vi "_convertDataPluginInfoToItems.vi"(8 "error in (no error)":errorcluster, 11 "DataPlugin information":T1[](array[typedef])) -> (0 "error out":errorcluster, 3 "Items":string[][](array[string]))   [LabVIEW 2020]
uses:
  <vilib>/Platform/storage/utility/DataPluginSynchronization/_DataPluginInfo.ctl
  <vilib>/Platform/storage/utility/DataPluginSynchronization/_localizeDataPluginMessageEnum.ctl
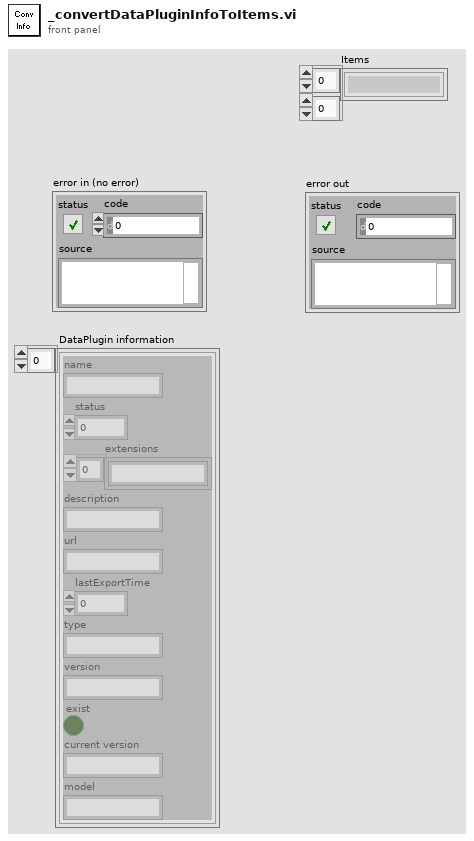
[diagram p1: front panel]
types:
  T1 = typedef "_DataPluginInfo.ctl" = cluster{"name":string, "status":u32, "extensions":string[], "description":string, "url":string, "lastExportTime":i64, "type":string, "version":string, "exist":bool, "current version":string, "model":string}
  T2 = typedef "_localizeDataPluginMessageEnum.ctl" = enum16{"Installed", "Not Installed", "Updates Available", "Latest version:", "Double click the \"Description\" cell.", "Install/Update DataPlugins", "Offline: ", "Please ensure that your network connection is working.", "No DataPlugins can be updated.", "Loading DataPlugins from ni.com/dataplugins", "Acquiring and installing ", "Install", "Update", "Succeed", "Failed", " Installation successful.", "Include *. to search for a file extension", "Current version:", " Installation failed.", "Installing update", "Update successful.", "Update failed.", "Updated", "Failed to update DataPlugins."}
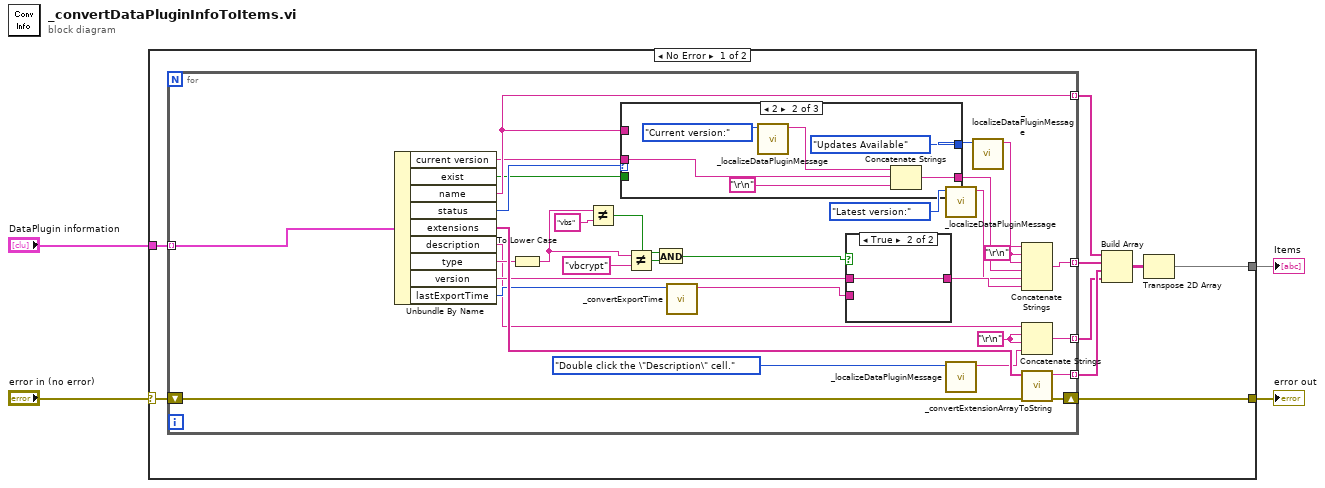
[diagram p0: block diagram]
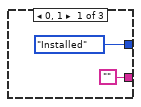
[diagram p3: hidden frame]
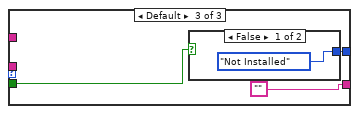
[diagram p4: hidden frame]
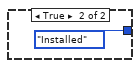
[diagram p5: hidden frame]
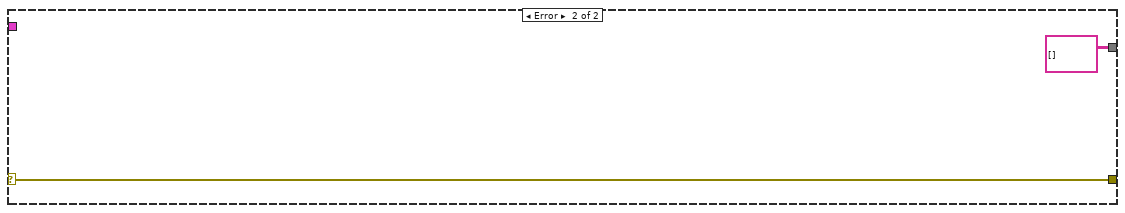
[diagram p6: hidden frame]
diagram:
  n1 = case shown="No Error" "error in (no error)" {
    selector: "error in (no error)" -> [w7 w62]
    tunnel: "DataPlugin information" -> [w5 _]
    tunnel: [w8 string[][] []] -> w4
    tunnel: [w6 w62] -> w2
    frame No Error {
      n2 = for {
        tunnel: w5 -> [w45] mode=indexing
        tunnel: [w18] -> w13 mode=indexing
        tunnel: [w28] -> w12 mode=indexing
        tunnel: [w43] -> w11 mode=indexing
        shift-right: [w41] -> w6
        shift-left: w7 -> [w42]
        tunnel: [w25] -> w10 mode=indexing
        w27 = "\r\n" ("string")
        w30 = "\r\n" ("string")
        n3 = Unbundle By Name(w45) -> ("current version"=w15:string, "exist"=w16:bool, "name"=w18:string, "status"=w40:u32, "extensions"=w44:string[], "description"=w26:string, "type"=w33:string, "version"=w32:string, "lastExportTime"=w39:i64)
        n4 = To Lower Case(string=w33) -> (all lower case string=w37:string)
        n5 = Not Equal?(x=w37, y="vbs") -> (x != y?=w35:bool)
        n6 = case shown="2" w40 {
          tunnel: [_localizeDataPluginMessageEnum."Installed" ("message in") _localizeDataPluginMessageEnum."Updates Available" ("message in") w58] -> w24
          tunnel: w18 -> [_ _ _]
          tunnel: w16 -> [_ _ w57]
          tunnel: w15 -> [_ w52 _]
          tunnel: ["" w50 ""] -> w14
          frame 0, 1 {
          }
          frame 2 {
            n7 = call <vilib>:"_localizeDataPluginMessage.vi"("message in"=_localizeDataPluginMessageEnum."Current version:") -> ("message out"=w53:string)  [unwired: 10 in]
            n8 = Concatenate Strings(w53, w52, "\r\n" ("string")) -> (w50:string)
          }
          frame Default {
            n9 = case shown="False" w57 {
              tunnel: [_localizeDataPluginMessageEnum."Not Installed" ("message in") _localizeDataPluginMessageEnum."Installed" ("message in")] -> w58
              frame False {
              }
              frame True {
              }
            }
          }
        }
        n10 = Not Equal?(x=w37, y="vbcrypt") -> (x != y?=w34:bool)
        n11 = And(x=w35, y=w34) -> (x .and. y?=w17:bool)
        n12 = call <vilib>:"_convertExportTime.vi"("lastExportTime"=w39) -> ("Time"=w31:string)  [unwired: 10 in]
        n13 = case shown="True" w17 {
          tunnel: w32 -> [_ w47]
          tunnel: w31 -> [w46 _]
          tunnel: [w46 w47] -> w29
          frame False {
          }
          frame True {
          }
        }
        n14 = call <vilib>:"_localizeDataPluginMessage.vi"("message in"=_localizeDataPluginMessageEnum."Latest version:") -> ("message out"=w21:string)  [unwired: 10 in]
        n15 = call <vilib>:"_localizeDataPluginMessage.vi"("message in"=_localizeDataPluginMessageEnum."Double click the \"Description\" cell.") -> ("message out"=w20:string)  [unwired: 10 in]
        n16 = call <vilib>:"_localizeDataPluginMessage.vi"("message in"=w24) -> ("message out"=w23:string)  [unwired: 10 in]
        n17 = Concatenate Strings(w23, w30, w30, w14, w21, w29) -> (w28:string)
        n18 = Concatenate Strings(w26, w27, w27, w20) -> (w25:string)
        n19 = call <vilib>:"_convertExtensionArrayToString.vi"("error in (no error)"=w42, "Extensions"=w44) -> ("error out"=w41:errorcluster, "Extension"=w43:string)  [unwired: 8 in]
      }
      n20 = Build Array(w13, w12, w11, w10) -> (w9:string[][])
      n21 = Transpose 2D Array(2D array=w9) -> (transposed array=w8:string[][])
    }
    frame Error {
    }
  }
  "Items" <- w4
  "error out" <- w2
